vi "Generate AO Sample Clock.vi"() -> ()   [LabVIEW 2009]
doc: "I. Description:\nThis example generates a clock of variable rate for the analog output circuitry. An array of 0V is the actual output, so the example is merely used to generate an analog clock.\n\nII. Instructions for Running:\n1. Select the Physical Channel to correspond to where an analog output channel on the DAQ device.\n2. Specify the desired Output Clock Rate (Hz). This control can be modified while the generation is taking place."
uses:
  <vilib>/DAQmx/write.llb/DAQmx Write (Analog 1D DBL 1Chan NSamp).vi
  <vilib>/DAQmx/configure/timing.llb/DAQmx Timing (Sample Clock).vi
  <vilib>/DAQmx/create/channels.llb/DAQmx Create Channel (AO-Voltage-Basic).vi
  Program Files/National Instruments/LabVIEW 2009/resource/objmgr/daqmx.rc
panel:
  in  "Output Clock Rate (Hz)":dbl(slide)=2.0 caption="Desired Frequency" scale=2.0..100.0
  in  "Physical Channels":tag
  in  "stop":bool
  # "Channel Parameters"
  # "Timing Parameters"
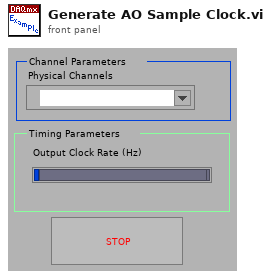
[diagram p1: front panel]
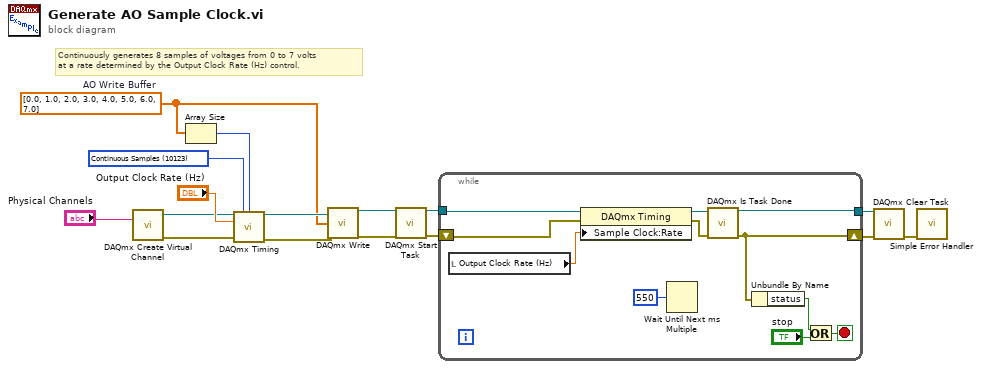
[diagram p0: block diagram]
diagram:
  w2 = dbl[] [0.0, 1.0, 2.0, 3.0, 4.0, 5.0, 6.0, 7.0]  # AO Write Buffer
  w15 = 10123 items=["Finite Samples"=10178, "Continuous Samples"=10123] ("sample mode")
  # "Continuously generates 8 samples of voltages from 0 to 7 volts\nat a rate determined by the Output Clock Rate (Hz) control."
  n1 = call-poly <vilib>:"DAQmx Create Virtual Channel.vi"("physical channels"="Physical Channels") -> ("task out"=w4:refnum<k21>, "error out"=w3:errorcluster)  [unwired: 13 in]
  n2 = Array Size(array=w2) -> (size(s)=w1:i32)
  n3 = call-poly <vilib>:"DAQmx Timing.vi"("task/channels in"=w4, "sample mode"=w15, "samples per channel"=w1, "rate"="Output Clock Rate (Hz)", "error in"=w3) -> ("task out"=w10:refnum<k21>, "error out"=w6:errorcluster)  [unwired: 9 in]
  n4 = call-poly <vilib>:"DAQmx Write.vi"("task/channels in"=w10, "data"=w2, "error in"=w6) -> ("task out"=w14:refnum<k21>, "error out"=w13:errorcluster)  [unwired: 10 in, 1 out]
  n5 = call <vilib>:"DAQmx Start Task.vi"("task/channels in"=w14, "error in"=w13) -> ("task out"=w16:refnum<k21>, "error out"=w12:errorcluster)  [unwired: 12 in]
  n6 = while {
    tunnel: w16 -> [w19]
    tunnel: [w22] -> w8
    shift-right: [w23] -> w7
    shift-left: w12 -> [w18]
    stop <- w27 stop-if-true
    n7 = local read "Output Clock Rate (Hz)"() -> (w17:dbl)
    n8 = property class="DAQmx Timing"(reference=w19, error in=w18, "Sample Clock:Rate"=w17) -> (reference out=w21:refnum<k21>, error out=w20:errorcluster)
    n9 = Wait Until Next ms Multiple(millisecond multiple=u32 550) -> ()  [unwired: 1 out]
    n10 = call <vilib>:"DAQmx Is Task Done.vi"("task/channels in"=w21, "error in"=w20) -> ("task out"=w22:refnum<k21>, "error out"=w23:errorcluster)  [unwired: 11 in, 1 out]
    n11 = Unbundle By Name(w23) -> ("status"=w25:bool)
    n12 = Or(x=w25, y="stop") -> (x .or. y?=w27:bool)
  }
  n13 = call <vilib>:"DAQmx Clear Task.vi"("task in"=w8, "error in"=w7) -> ("error out"=w9:errorcluster)  [unwired: 13 in]
  n14 = call <vilib>:"Simple Error Handler.vi"("error in (no error)"=w9) -> ()  [unwired: 4 in, 5 out]
